vi "ev Apply change.vi"(8 "error in (no error)":errorcluster, 11 "IDE simple in":refnum<class "LF2R IDE.lvclass">) -> (0 "error out":errorcluster, 3 "IDE simple out":refnum<class "LF2R IDE.lvclass">)   [LabVIEW 2018, in "LF2R IDE.lvlib" / "LF2R IDE.lvclass"]
uses:
  LF2R IDE.lvclass
  LF2R IDE.lvclass/LF2R IDE.ctl
  Frame Analizer/Data Parser.lvclass
  ScintillaNET/ScintillaNET.lvclass
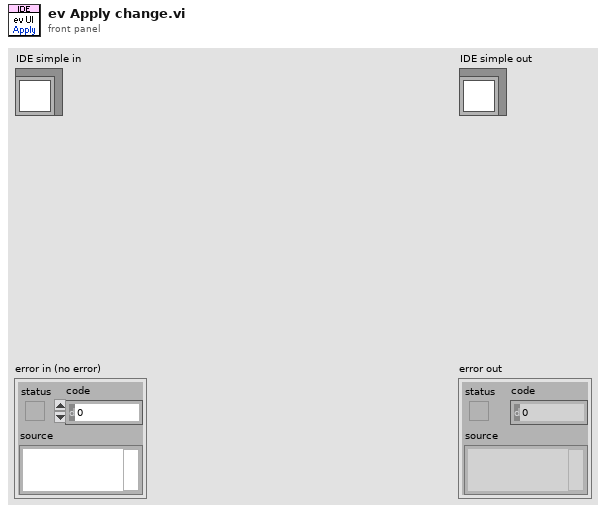
[diagram p1: front panel]
types:
  T1 = typedef "Data Parser.lvclass/frame data.ctl" = cluster{"Title":T2, "Basic Data":T3, "Sound":string, "<o> Data":T4, "<bp> Data":T5, "<c> Data":T6, "<w> Data":T7, "<i> Data Array":T8[], "<b> Data Array":T9[]}
  T2 = typedef "Data Parser.lvclass/frame title.ctl" = cluster{"number":string, "name":string}
  T3 = typedef "Data Parser.lvclass/frame basic data.ctl" = cluster{"Basic":cluster{"pic":string, "state":string, "wait":string, "next":string}, "Move":cluster{"dvx":string, "dvy":string, "dvz":string}, "Pic Center":cluster{"centerx":string, "centery":string}, "Skill":cluster{"hit_a":string, "hit_d":string, "hit_j":string, "hit_Fa":string, "hit_Ua":string, "hit_Da":string, "hit_Fj":string, "hit_Uj":string, "hit_Dj":string, "hit_ja":string}, "Mp":string}
  T4 = typedef "Data Parser.lvclass/frame o data.ctl" = cluster{"kind":string, "x":string, "y":string, "action":string, "dvx":string, "dvy":string, "dvz":string, "oid":string, "facing":string}
  T5 = typedef "Data Parser.lvclass/frame bp data.ctl" = cluster{"x":string, "y":string}
  T6 = typedef "Data Parser.lvclass/frame c data.ctl" = cluster{"kind":string, "x":string, "y":string, "injury":string, "cover":string, "vaction":string, "aaction":string, "taction":string, "hurtable":string, "decrease":string, "fronthurtact":string, "backhurtact":string, "dircontrol":string, "throwvx":string, "throwvy":string, "throwvz":string, "throwinjury":string}
  T7 = typedef "Data Parser.lvclass/frame w data.ctl" = cluster{"kind":string, "x":string, "y":string, "weaponact":string, "dvx":string, "dvy":string, "dvz":string, "attacking":string, "cover":string}
  T8 = typedef "Data Parser.lvclass/frame i data.ctl" = cluster{"kind":string, "x":string, "y":string, "w":string, "h":string, "dvx":string, "dvy":string, "dvz":string, "fall":string, "arest":string, "vrest":string, "bdefend":string, "injury":string, "zwidth":string, "effect":string, "catchingact":string, "caughtact":string}
  T9 = typedef "Data Parser.lvclass/frame b data.ctl" = cluster{"kind":string, "x":string, "y":string, "w":string, "h":string}
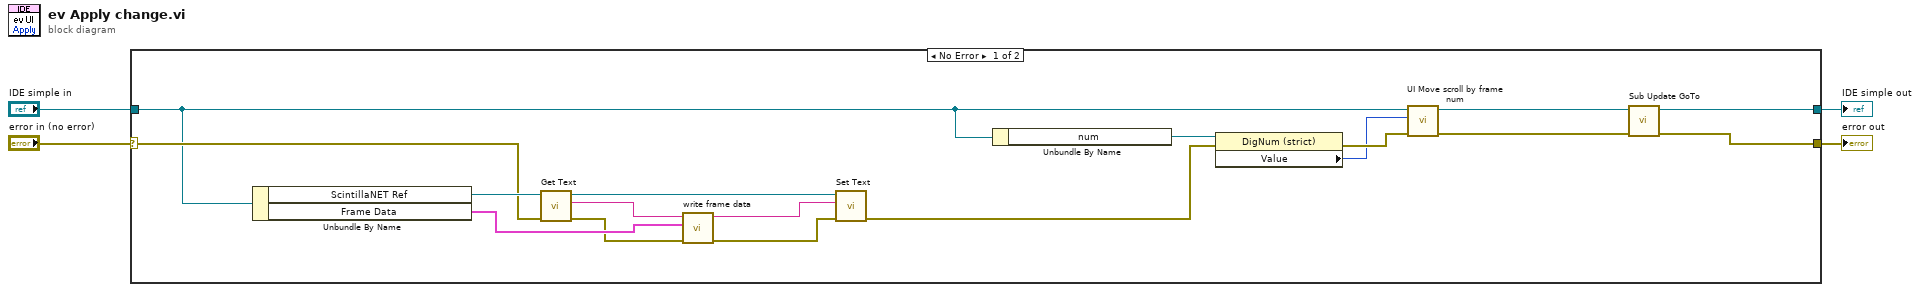
[diagram p0: block diagram]
diagram:
  n1 = case shown="No Error" "error in (no error)" {
    selector: "error in (no error)" -> [w14 w23]
    tunnel: [w5 w23] -> w3
    tunnel: [w6 w22] -> w1
    tunnel: "IDE simple in" -> [w12 w22]
    frame No Error {
      n2 = Unbundle By Name(w12) -> ("ScintillaNET Ref"=w20:refnum<class "ScintillaNET.lvclass">, "Frame Data"=w21:T1)
      n3 = call "Get Text.vi"("error in (no error)"=w14, "ScintillaNET in"=w20) -> ("error out"=w18:errorcluster, "Text"=w19:string, "ScintillaNET out"=w16:refnum<class "ScintillaNET.lvclass">)  [unwired: 7 in]
      n4 = call "write frame data.vi"("error in"=w18, "frame data"=w21, "file string in"=w19) -> ("error out"=w17:errorcluster, "file string out"=w15:string)  [unwired: 7 in]
      n5 = call "Set Text.vi"("error in (no error)"=w17, "Text"=w15, "ScintillaNET in"=w16) -> ("error out"=w11:errorcluster)  [unwired: 7 in, 1 out]
      n6 = Unbundle By Name(w12) -> ("num"=w13:refnum<vi>)
      n7 = property class="DigNum (strict)"(reference=w13, error in=w11) -> (error out=w10:errorcluster, "Value"=w9:u32)  [unwired: 1 out]
      n8 = call "UI Move scroll by frame num.vi"("error in (no error)"=w10, "frame number"=w9, "IDE simple in"=w12) -> ("error out"=w7:errorcluster, "IDE simple out"=w8:refnum<class "LF2R IDE.lvclass">)  [unwired: 7 in]
      n9 = call "Sub Update GoTo.vi"("error in (no error)"=w7, "LF2R IDE in"=w8) -> ("error out"=w5:errorcluster, "LF2R IDE out"=w6:refnum<class "LF2R IDE.lvclass">)  [unwired: 8 in]
    }
    frame Error {
    }
  }
  "error out" <- w3
  "IDE simple out" <- w1
